vi "HFRR ADV v10.vi"() -> ()   [LabVIEW 2025] (continued)
                    n423 = Fract/Exp String To Number(string=w685) -> (number=w684:dbl)  [unwired: 3 in, 1 out]
                    n424 = local write "Average"(w684) -> ()
                  }
                }
              }
              frame True {
                w723 = 1000.0 ("y")
                w729 = 0.0 ("default (0 DBL)")
                n425 = Match Pattern(string=w735, regular expression=" \"width_px\":") -> (after substring=w733:string)  [unwired: 1 in, 3 out]
                n426 = Match Pattern(string=w733, regular expression="\"height_px\":") -> (before substring=w731:string, after substring=w730:string)  [unwired: 1 in, 2 out]
                n427 = Fract/Exp String To Number(string=w731, default (0 dbl)=w729) -> (number=w728:dbl)  [unwired: 2 in, 1 out]
                n428 = Fract/Exp String To Number(string=w730, default (0 dbl)=w729) -> (number=w727:dbl)  [unwired: 2 in, 1 out]
                n429 = Multiply(x=w728, y=w726) -> (x*y=w725:dbl)
                n430 = Multiply(x=w727, y=w726) -> (x*y=w724:dbl)
                n431 = Multiply(x=w725, y=w723) -> (x*y=w709:dbl)
                n432 = Multiply(x=w724, y=w723) -> (x*y=w707:dbl)
                n433 = Add(x=w709, y=w707) -> (x+y=w721:dbl)
                n434 = property on="Major Axis" class="DigNum (strict)"("Caption.Text"="Major Axis") -> ()  [unwired: 2 in, 2 out]
                n435 = property on="Minor Axis" class="DigNum (strict)"("Caption.Text"="Minor Axis") -> ()  [unwired: 2 in, 2 out]
                n436 = property on="Average" class="DigNum (strict)"("Caption.Text"="Average") -> ()  [unwired: 2 in, 2 out]
                n437 = Divide(x=w721, y=2.0) -> (x/y=w705:dbl)
                n438 = Bundle By Name(cluster=w722, "major"=w709, "minor"=w707, "average"=w705) -> (w719:cluster{"major":dbl, "minor":dbl, "average":dbl})
                n439 = Number To Fractional String(number=w707, precision (6)=i16 1) -> (F-format string=w714:string)  [unwired: 2 in]
                n440 = Number To Fractional String(number=w705, precision (6)=i16 1) -> (F-format string=w715:string)  [unwired: 2 in]
                n441 = Number To Fractional String(number=w709, precision (6)=i16 1) -> (F-format string=w713:string)  [unwired: 2 in]
                n442 = Fract/Exp String To Number(string=w714) -> (number=w706:dbl)  [unwired: 3 in, 1 out]
                n443 = Fract/Exp String To Number(string=w715) -> (number=w704:dbl)  [unwired: 3 in, 1 out]
                n444 = Fract/Exp String To Number(string=w713) -> (number=w708:dbl)  [unwired: 3 in, 1 out]
                n445 = local write "Major Axis"(w708) -> ()
                n446 = local write "Average"(w704) -> ()
                n447 = local write "Minor Axis"(w706) -> ()
              }
            }
            n448 = case shown="\"Measrument\", Default" w622 {
              tunnel: w625 -> [w649 _]
              tunnel: w624 -> [w648 _]
              tunnel: [w645 w673] -> w623
              tunnel: w621 -> [w647 w673]
              tunnel: w620 -> [w646 _]
              frame "Measrument", Default {
                n449 = stacked-sequence {
                  tunnel: w649 -> [w666 _]
                  tunnel: w648 -> [w664 _]
                  tunnel: w647 -> [w662 _]
                  tunnel: w646 -> [w661 _]
                  tunnel: [w656 _] -> w645
                  frame #0 {
                    n450 = call "IMAGE ANALYSIS.vi"("Enum"=POST_ANALYSIS_ENUM."SAVE IMAGE", "error in"=w662, "IMAGE FILE PATH"=w661) -> ("error out"=w660:errorcluster)  [unwired: 7 in, 1 out]
                    n451 = call "Stall Data Flow.vim"("value in"=w660, "milliseconds to wait"=u32 1000) -> ("value out"=w651:errorcluster)  [unwired: 1 out]
                    n452 = local read "Test File List :"() -> (w668:string)
                    n453 = call "IMAGE ANALYSIS.vi"("Enum"=POST_ANALYSIS_ENUM."MINIMIZE UI", "error in"=w651) -> ("error out"=w658:errorcluster)  [unwired: 8 in, 1 out]
                    n454 = Bundle By Name(cluster=T21 {"File Name"="", "Test Method"="", "Operator"="", "Fuel Description"="", "Date and time"=""} ("Main Ref"), "File Name"=w668) -> (w669:T21)
                    n455 = call "Stall Data Flow.vim"("value in"=w658, "milliseconds to wait"=u32 1500) -> ("value out"=w653:errorcluster)  [unwired: 1 out]
                    n456 = call "duf file read.vi"("error in (no error)"=w653, "Main Ref"=w669) -> ("error out"=w667:errorcluster, "Main Ref 2"=w665:T21)  [unwired: 8 in]
                    n457 = call "DETECTION REPORT for manual.vi"("error in (no error)"=w667, "return value 3"=w664, "Image File Path"=w666, "Main Ref"=w665) -> ("error out"=w663:errorcluster)  [unwired: 7 in]
                    n458 = call <vilib>:"Clear Errors.vi"("error in (no error)"=w663) -> ("error out"=w654:errorcluster)  [unwired: 5 in, 1 out]
                    n459 = call "IMAGE ANALYSIS.vi"("Enum"=POST_ANALYSIS_ENUM."MINIMIZE UI", "error in"=w654) -> ("error out"=w656:errorcluster)  [unwired: 8 in, 1 out]
                  }
                  frame #1 {
                    n460 = local write "Main Tab"(T2."HOME" ("Main Tab")) -> ()
                    n461 = local write "Main Dashboard Buttons"(T1."Home" ("Main Dashboard Buttons")) -> ()
                  }
                }
              }
              frame "Calibrate" {
              }
            }
          }
          frame #2 {
            n462 = Not(x=w738) -> (.not. x?=w737:bool)
            n463 = local write "Confirm Measrurement"(w737) -> ()
            n464 = local read "Calibration Tab"() -> (w736:enum32{"Measrument", "Calibrate"})
            n465 = case shown="\"Measrument\", Default" w736 {
              frame "Measrument", Default {
                n466 = local write "Main Tab"(T2."HOME" ("Main Tab")) -> ()
              }
              frame "Calibrate" {
              }
            }
          }
        }
      }
    }
    n467 = local read "Humidity"() -> (w487:bool)
    n468 = local read "Save Change"() -> (w492:bool)
    n469 = local read "Calibrate"() -> (w493:bool)
    n470 = local read "Auto Start Test"() -> (w488:bool)
    n471 = case shown="True" w493 {
      selector: w493 -> [_ w600]
      frame False {
      }
      frame True {
        n472 = Not(x=w600) -> (.not. x?=w599:bool)
        n473 = local write "Calibrate"(w599) -> ()
        n474 = local write "Calibration Tab"(enum32{"Measrument", "Calibrate"}."Calibrate" ("Calibration Tab")) -> ()
      }
    }
    n475 = case shown="True" w492 {
      selector: w492 -> [_ w544]
      frame False {
      }
      frame True {
        n476 = stacked-sequence {
          tunnel: w544 -> [_ _ _ _ w598]
          frame #0 {
            n477 = call "IMAGE ANALYSIS.vi"("Enum"=POST_ANALYSIS_ENUM."HIDE UI") -> ()  [unwired: 9 in, 2 out]
          }
          frame #1 {
            n478 = local read "100x gain"() -> (w546:dbl)
            n479 = local read "10x Gain"() -> (w547:dbl)
            n480 = local read "5x Gain"() -> (w548:dbl)
            n481 = Number To Fractional String(number=w547, width (-)=i16 4, precision (6)=i16 7) -> (F-format string=w569:string)  [unwired: 1 in]
            n482 = Number To Fractional String(number=0.0, width (-)=i16 4, precision (6)=i16 7) -> (F-format string=w564:string)  [unwired: 1 in]
            n483 = Number To Fractional String(number=w546, width (-)=i16 4, precision (6)=i16 7) -> (F-format string=w552:string)  [unwired: 1 in]
            n484 = Number To Fractional String(number=w548, width (-)=i16 10 ("precision (6)"), precision (6)=i16 7) -> (F-format string=w578:string)  [unwired: 1 in]
            n485 = Concatenate Strings("[CH1]" ("string"), w578, " - 5x Gain" ("string"), "\r") -> (w568:string)
            n486 = Concatenate Strings("[CH2]" ("string"), w569, " - 10x Gain" ("string"), "\r") -> (w567:string)
            n487 = Concatenate Strings("[CH3]" ("string"), w564, " - 20x Gain" ("string"), "\r") -> (w558:string)
            n488 = Concatenate Strings("[CH4]" ("string"), w552, " - 100x Gain" ("string"), "\r") -> (w551:string)
            n489 = String To Path(string="C:\\LAB-IQ\\Image Calibrate v01.dcf") -> (path=w581:path)
            n490 = Concatenate Strings(w568, w567, w558, w551) -> (w566:string)
            n491 = call <vilib>:"Write Characters To File.vi"("append to file? (new file:F)"=FALSE, "character string"=w566, "file path (dialog if empty)"=w581) -> ()  [unwired: 2 in, 1 out]
          }
          frame #2 {
            n492 = String To Path(string="C:\\LAB-IQ\\Image Calibrate v01.dcf") -> (path=w584:path)
            n493 = Open/Create/Replace File ("Open File")(file path (use dialog)=w584) -> (refnum out=w585:refnum<file>)  [unwired: 5 in, 2 out]
            n494 = for {
              N: 4 -> [_]
              tunnel: w585 -> [w591]
              i -> [w587]
              n495 = Read from Text File ("Read File")(file (use dialog)=w591) -> (text=w592:string)  [unwired: 3 in, 3 out]
              n496 = String Subset(string=w592, offset (0)=6, length (rest)=10 ("length (rest)")) -> (substring=w588:string)
              n497 = Fract/Exp String To Number(string=w588) -> (number=w586:dbl)  [unwired: 3 in, 1 out]
              n498 = case shown="3" w587 {
                tunnel: w586 -> [w593 w594 _ w595 _]
                frame 0 {
                  n499 = local write "5x Gain"(w593) -> ()
                }
                frame 1 {
                  n500 = local write "10x Gain"(w594) -> ()
                }
                frame 2 {
                }
                frame 3 {
                  n501 = local write "100x gain"(w595) -> ()
                }
                frame 4, Default {
                }
              }
            }
          }
          frame #3 {
            n502 = call "IMAGE ANALYSIS.vi"("Enum"=POST_ANALYSIS_ENUM."SHOW UI") -> ()  [unwired: 9 in, 2 out]
          }
          frame #4 {
            n503 = Not(x=w598) -> (.not. x?=w597:bool)
            n504 = local write "Save Change"(w597) -> ()
          }
        }
      }
    }
    n505 = case shown="False" w488 {
      tunnel: w487 -> [w514 _]
      frame False {
        n506 = case shown="True" w514 {
          frame False {
          }
          frame True {
            n507 = local read "Set Humidity:"() -> (w518:dbl)
            n508 = local read "Set Humidity:"() -> (w521:dbl)
            n509 = local read "Humidity ( %RH )"() -> (w522:dbl)
            n510 = Subtract(x=w518, y=1.0) -> (x-y=w516:dbl)
            n511 = Add(x=w521, y=1.0) -> (x+y=w517:dbl)
            n512 = In Range and Coerce(upper limit=w517, x=w522, lower limit=w516) -> (In Range?=w515:bool)  [unwired: 1 out]
            n513 = case shown="True" w515 {
              frame False {
              }
              frame True {
                n514 = case shown="True" "Manual Humididty Reached" {
                  selector: "Manual Humididty Reached" -> [_ w525]
                  frame False {
                  }
                  frame True {
                    n515 = Not(x=w525) -> (.not. x?=w524:bool)
                    n516 = local write "Manual Humididty Reached"(w524) -> ()
                    n517 = local read "EVENT LOG"() -> (w527:string)
                    n518 = call "Event Log.vi"("Content"="Target Humidity reached", "EVENT LOG"=w527) -> ("EVENT LOG"=w526:string)  [unwired: 8 in, 1 out]
                    n519 = local write "EVENT LOG"(w526) -> ()
                  }
                }
              }
            }
          }
        }
      }
      frame True {
        n520 = local write "Manual Humididty Reached"(TRUE ("Manual Humididty Reached")) -> ()
      }
    }
    n521 = local read "Cap Live Image"() -> (w508:bool)
    n522 = local read "SCAR MEASURMENT"() -> (w511:enum32{"Auto Scar", "Manual Scar"})
    n523 = Wait (ms)(milliseconds to wait=u32 250) -> ()  [unwired: 1 out]
    n524 = Equal?(x=w511, y=enum32{"Auto Scar", "Manual Scar"}."Manual Scar" ("SCAR MEASURMENT")) -> (x = y?=w509:bool)
    n525 = And(x=w509, y=w508) -> (x .and. y?=w507:bool)
    n526 = case shown="True" w507 {
      selector: w507 -> [_ w817]
      frame False {
      }
      frame True {
        n527 = stacked-sequence {
          tunnel: [_ _ _ w832 _] -> _
          tunnel: w817 -> [_ _ _ _ w838]
          frame #0 {
            w818 = 0.0
            n528 = local write "Major Axis"(w818) -> ()
            n529 = local write "Minor Axis"(w818) -> ()
            n530 = local write "Average"(w818) -> ()
          }
          frame #1 {
            n531 = call "CAMERA LIVE FEED FGV.vi"("Enum - Menu"=CAMERA_LIVE_FEED_ENUM."CAMERA MINIMIZE") -> ()  [unwired: 9 in, 2 out]
          }
          frame #2 {
            n532 = local read "FILE 3"() -> (w826:string)
            n533 = call <vilib>:"Trim Whitespace.vi"("string"="C:\\LAB-IQ\\images\\") -> ("trimmed string"=w828:string)  [unwired: 1 in]
            n534 = String To Path(string=w828) -> (path=w827:path)
            n535 = Concatenate Strings(w826, ".png" ("string")) -> (w825:string)
            n536 = Build Path(base path=w827, name or relative path=w825) -> (appended path=w823:path)
            n537 = Path To String(path=w823) -> (string=w822:string)
            n538 = call "CAMERA LIVE FEED FGV.vi"("Enum - Menu"=CAMERA_LIVE_FEED_ENUM."CAMERA SAVE", "Image Path"=w822) -> ("error out"=w820:errorcluster)  [unwired: 8 in, 1 out]
            n539 = case shown="No Error" w820 {
              frame No Error {
                n540 = One Button Dialog(message="Image saved successfully") -> ()  [unwired: 1 in, 1 out]
              }
              frame Error {
              }
            }
          }
          frame #3 {
            n541 = call "LIST FILE NAMES.vi"() -> ("error out"=w834:errorcluster, "filenames"=w831:string[])  [unwired: 10 in]
            n542 = call "IMAGE ANALYSIS.vi"("Enum"=POST_ANALYSIS_ENUM."SHOW UI", "error in"=w834) -> ("error out"=w832:errorcluster)  [unwired: 8 in, 1 out]
            n543 = property on="Test File List :" class="CmbBox"("Strings[]"=w831) -> ()  [unwired: 2 in, 2 out]
          }
          frame #4 {
            (unwired) T22."Report" ("Main Dashboard Buttons")
            n544 = Not(x=w838) -> (.not. x?=w837:bool)
            n545 = local write "Zoom Factore"(0.0 ("Zoom Factore")) -> ()
            n546 = local write "Cap Live Image"(w837) -> ()
            n547 = local write "Main Tab"(T2."Adv Scar Report" ("Main Tab")) -> ()
            n548 = property on="Cap Live Image" class="Bool (strict)"("BoolText.Text"="Capture Image" ("Boolean Text.Text")) -> ()  [unwired: 2 in, 2 out]
            n549 = local write "Main Dashboard Buttons"(T1."Report" ("Main Dashboard Buttons")) -> ()
          }
        }
      }
    }
    n550 = local read "change Gain"() -> (w491:bool)
    n551 = local read "Back Square"() -> (w490:bool)
    n552 = case shown="True" w491 {
      selector: w491 -> [_ w535]
      frame False {
      }
      frame True {
        n553 = stacked-sequence {
          tunnel: w535 -> [_ w543]
          frame #0 {
            n554 = local read "Actual (µm)"() -> (w539:dbl)
            n555 = local read "Pixel Value"() -> (w538:dbl)
            n556 = local read "Magnification :"() -> (w537:string)
            n557 = Divide(x=w539, y=w538) -> (x/y=w536:dbl)
            n558 = case shown="\"10x\"" w537 {
              tunnel: w536 -> [w540 w541]
              frame "10x" {
                n559 = local write "10x Gain"(w540) -> ()
              }
              frame "5x", Default {
                n560 = local write "5x Gain"(w541) -> ()
              }
            }
          }
          frame #1 {
            n561 = Not(x=w543) -> (.not. x?=w542:bool)
            n562 = local write "change Gain"(w542) -> ()
          }
        }
      }
    }
    n563 = case shown="True" w490 {
      selector: w490 -> [_ w533]
      frame False {
      }
      frame True {
        n564 = Not(x=w533) -> (.not. x?=w532:bool)
        n565 = local write "Back Square"(w532) -> ()
        n566 = local write "Calibration Tab"(enum32{"Measrument", "Calibrate"}."Measrument" ("Calibration Tab")) -> ()
      }
    }
    n567 = local read "Rectangle Tool"() -> (w502:bool)
    n568 = local read "Clear ROI Tool"() -> (w501:bool)
    n569 = local read "Open Image"() -> (w506:bool)
    n570 = local read "line tool"() -> (w503:bool)
    n571 = local read "OUT"() -> (w504:bool)
    n572 = local read "In"() -> (w505:bool)
    n573 = case shown="True" w506 {
      selector: w506 -> [_ w805]
      tunnel: [w801 w807] -> _
      tunnel: w496 -> [w801 w806]
      frame False {
      }
      frame True {
        n574 = Not(x=w805) -> (.not. x?=w804:bool)
        n575 = local write "Open Image"(w804) -> ()
        n576 = call "IMAGE ANALYSIS.vi"("Enum"=POST_ANALYSIS_ENUM."HIDE UI", "error in"=w806) -> ("error out"=w814:errorcluster)  [unwired: 8 in, 1 out]
        n577 = call "File Dialog"("start path"=path "C:/LAB-IQ/images", "error in"=w814) -> ("selected path"=w803:path, "error out"=w812:errorcluster)  [unwired: 10 in, 2 out]
        "Image path  2" <- w803
        n578 = call <vilib>:"Clear Errors.vi"("error in (no error)"=w812) -> ("error out"=w811:errorcluster)  [unwired: 5 in, 1 out]
        n579 = call "IMAGE ANALYSIS.vi"("Enum"=POST_ANALYSIS_ENUM."OPEN FILE", "error in"=w811, "File Path"=w803) -> ("error out"=w810:errorcluster)  [unwired: 7 in, 1 out]
        n580 = call <vilib>:"Clear Errors.vi"("error in (no error)"=w810) -> ("error out"=w809:errorcluster)  [unwired: 5 in, 1 out]
        n581 = call "IMAGE ANALYSIS.vi"("Enum"=POST_ANALYSIS_ENUM."SHOW UI", "error in"=w809) -> ("error out"=w807:errorcluster)  [unwired: 8 in, 1 out]
        n582 = local write "Zoom Factore"(100.0 ("Zoom Factore")) -> ()
      }
    }
    n583 = case shown="True" w504 {
      selector: w504 -> [_ w786]
      tunnel: w496 -> [w783 w791]
      tunnel: [w783 w785] -> _
      frame False {
      }
      frame True {
        n584 = Not(x=w786) -> (.not. x?=w784:bool)
        n585 = local read "Zoom Factore"() -> (w789:dbl)
        n586 = local write "OUT"(w784) -> ()
        n587 = call "IMAGE ANALYSIS.vi"("Enum"=POST_ANALYSIS_ENUM."ZOOM OUT", "error in"=w791) -> ("error out"=w785:errorcluster)  [unwired: 8 in, 1 out]
        n588 = Divide(x=w789, y=1.2) -> (x/y=w787:dbl)
        n589 = local write "Zoom Factore"(w787) -> ()
      }
    }
    n590 = case shown="True" w505 {
      selector: w505 -> [_ w795]
      tunnel: w496 -> [w792 w800]
      tunnel: [w792 w793] -> _
      frame False {
      }
      frame True {
        n591 = Not(x=w795) -> (.not. x?=w794:bool)
        n592 = local read "Zoom Factore"() -> (w798:dbl)
        n593 = local write "In"(w794) -> ()
        n594 = call "IMAGE ANALYSIS.vi"("Enum"=POST_ANALYSIS_ENUM."ZOOM IN", "error in"=w800) -> ("error out"=w793:errorcluster)  [unwired: 8 in, 1 out]
        n595 = Multiply(x=w798, y=1.2) -> (x*y=w796:dbl)
        n596 = local write "Zoom Factore"(w796) -> ()
      }
    }
    n597 = case shown="True" w501 {
      selector: w501 -> [_ w767]
      tunnel: w496 -> [w765 w769]
      tunnel: [w765 w768] -> _
      frame False {
      }
      frame True {
        n598 = Not(x=w767) -> (.not. x?=w766:bool)
        n599 = local write "Clear ROI Tool"(w766) -> ()
        n600 = call "IMAGE ANALYSIS.vi"("Enum"=POST_ANALYSIS_ENUM."CLEAR ROI", "error in"=w769) -> ("error out"=w768:errorcluster)  [unwired: 8 in, 1 out]
      }
    }
    n601 = case shown="True" w503 {
      selector: w503 -> [_ w779]
      tunnel: w496 -> [w777 w782]
      tunnel: [w777 w780] -> _
      frame False {
      }
      frame True {
        n602 = Not(x=w779) -> (.not. x?=w778:bool)
        n603 = local write "line tool"(w778) -> ()
        n604 = call "IMAGE ANALYSIS.vi"("Enum"=POST_ANALYSIS_ENUM."DRAW LINE", "error in"=w782) -> ("error out"=w780:errorcluster)  [unwired: 8 in, 1 out]
      }
    }
    n605 = case shown="True" w502 {
      selector: w502 -> [_ w773]
      tunnel: w496 -> [w771 w775]
      tunnel: [w771 w774] -> _
      frame False {
      }
      frame True {
        n606 = Not(x=w773) -> (.not. x?=w772:bool)
        n607 = local write "Rectangle Tool"(w772) -> ()
        n608 = call "IMAGE ANALYSIS.vi"("Enum"=POST_ANALYSIS_ENUM."DRAW REC", "error in"=w775) -> ("error out"=w774:errorcluster)  [unwired: 8 in, 1 out]
      }
    }
    n609 = local read "SCAR MEASURMENT"() -> (w489:enum32{"Auto Scar", "Manual Scar"})
    n610 = local read "Fit to Screen Tool"() -> (w498:bool)
    n611 = local read "Resize Tool"() -> (w497:bool)
    n612 = case shown="\"Manual Scar\", Default" w489 {
      frame "Auto Scar" {
        n613 = property on="Cap Live Image" class="Bool (strict)"("BoolText.Text"="Report" ("Boolean Text.Text")) -> ()  [unwired: 2 in, 2 out]
      }
      frame "Manual Scar", Default {
        n614 = property on="Cap Live Image" class="Bool (strict)"("BoolText.Text"="Save Image" ("Boolean Text.Text")) -> ()  [unwired: 2 in, 2 out]
      }
    }
    n615 = local read "ROI Color Tool"() -> (w499:bool)
    n616 = local read "Pan Tool"() -> (w500:bool)
    n617 = case shown="True" w500 {
      selector: w500 -> [_ w761]
      tunnel: w496 -> [w759 w763]
      tunnel: [w759 w762] -> _
      frame False {
      }
      frame True {
        n618 = Not(x=w761) -> (.not. x?=w760:bool)
        n619 = call "IMAGE ANALYSIS.vi"("Enum"=POST_ANALYSIS_ENUM."PAN", "error in"=w763) -> ("error out"=w762:errorcluster)  [unwired: 8 in, 1 out]
        n620 = local write "Pan Tool"(w760) -> ()
      }
    }
    n621 = case shown="True" w497 {
      selector: w497 -> [_ w745]
      tunnel: w496 -> [w740 w742]
      tunnel: [w740 w741] -> _
      frame False {
      }
      frame True {
        n622 = Not(x=w745) -> (.not. x?=w744:bool)
        n623 = local write "Resize Tool"(w744) -> ()
        n624 = call "IMAGE ANALYSIS.vi"("Enum"=POST_ANALYSIS_ENUM."RESIZE MODE", "error in"=w742) -> ("error out"=w741:errorcluster)  [unwired: 8 in, 1 out]
      }
    }
    n625 = case shown="True" w498 {
      selector: w498 -> [_ w750]
      tunnel: [w746 w751] -> _
      tunnel: w496 -> [w746 w749]
      frame False {
      }
      frame True {
        n626 = Not(x=w750) -> (.not. x?=w748:bool)
        n627 = local write "Zoom Factore"(100.0 ("Zoom Factore")) -> ()
        n628 = local write "Fit to Screen Tool"(w748) -> ()
        n629 = call "IMAGE ANALYSIS.vi"("Enum"=POST_ANALYSIS_ENUM."FIT", "error in"=w749) -> ("error out"=w751:errorcluster)  [unwired: 8 in, 1 out]
      }
    }
    n630 = case shown="True" w499 {
      selector: w499 -> [_ w756]
      tunnel: [w753 w757] -> _
      tunnel: w496 -> [w753 w754]
      frame False {
      }
      frame True {
        n631 = Not(x=w756) -> (.not. x?=w755:bool)
        n632 = local write "ROI Color Tool"(w755) -> ()
        n633 = call "IMAGE ANALYSIS.vi"("Enum"=POST_ANALYSIS_ENUM."SET ROI COLOR", "error in"=w754) -> ("error out"=w757:errorcluster)  [unwired: 8 in, 1 out]
      }
    }
    n634 = local read "Quit"() -> (w513:bool)
  }
  n635 = local write "USERNAME"(w28) -> ()
  n636 = local write "Main Tab"(T2."HOME" ("Main Tab")) -> ()
  n637 = local write "USER ID"(w28) -> ()
  n638 = property on="Auto Scar Check  2" class="Clust (strict)"("Visible"=w9) -> (error out=w13:errorcluster)  [unwired: 2 in, 1 out]
  n639 = property on="Quit" class="Bool (strict)"("Value"=FALSE ("Quit")) -> (error out=w30:errorcluster)  [unwired: 2 in, 1 out]
  n640 = while {
    stop <- w841 stop-if-true
    n641 = local read "Image Path"() -> (w844:path)
    n642 = local read "Print 3"() -> (w847:bool)
    n643 = Equal?(x=w844, y=path "") -> (x = y?=w843:bool)
    n644 = Not(x=w843) -> (.not. x?=w842:bool)
    n645 = property on="Print 3" class="Bool (strict)"("Visible"=w842) -> ()  [unwired: 2 in, 2 out]
    n646 = case shown="True" w847 {
      frame False {
        n647 = local write "Rd"(TRUE ("Boolean 7")) -> ()
      }
      frame True {
        n648 = flat-sequence {
          tunnel: [w887] -> w855
          tunnel: [w874] -> w853
          tunnel: [w884] -> w849
          tunnel: w855 -> [w896]
          tunnel: [w896] -> w854
          tunnel: w853 -> [w895]
          tunnel: [w895] -> w852
          tunnel: [w893] -> w851
          tunnel: [w892] -> w850
          tunnel: w849 -> [w892]
          tunnel: w854 -> [w898]
          tunnel: w852 -> [w899]
          tunnel: w851 -> [_]
          tunnel: w850 -> [w897]
          frame #0 {
            n649 = case shown="True" "Rd" {
              frame False {
              }
              frame True {
                n650 = while {
                  tunnel: "abcdefABCDEF" ("string 2") -> [w866]
                  shift-right: [w864] -> w858
                  shift-left: "" -> [w863]
                  i -> [w873]
                  stop <- w872 stop-if-true
                  n651 = Random Number (0-1)() -> (number: 0 to 1=w867:dbl)
                  n652 = Multiply(x=w867, y=62.0) -> (x*y=w869:dbl)
                  n653 = Decrement(x="Length 2") -> (x-1=w862:i16)
                  n654 = To Word Integer(number=w869) -> (16bit integer=w870:i16)
                  n655 = String Subset(string=w866, offset (0)=w870, length (rest)=1 ("length (rest)")) -> (substring=w865:string)
                  n656 = Greater Or Equal?(x=w873, y=w862) -> (x >= y?=w872:bool)
                  n657 = Concatenate Strings(w865, w863) -> (w864:string)
                }
                "String 10" <- w858
                n658 = local write "Rd"(FALSE ("Boolean 7")) -> ()
              }
            }
          }
          frame #1 {
            w885 = "_resized.jpg" ("command line")
            (unwired) ".jpg -resize 320x240 " ("string")
            (unwired) "Choose an Image File" ("prompt")
            # "-resize 1798x425"
            n659 = local read "Image Path"() -> (w879:path)
            n660 = Strip Path(path=w879) -> (stripped path=w874:path, name=w875:string)
            n661 = Match Pattern(string=w875, regular expression=".jpg") -> (before substring=→"before substring 2":string, after substring=→"after substring":string)  [unwired: 1 in, 2 out]
            n662 = Match Pattern(string=w875, regular expression="\\") -> (before substring=w881:string)  [unwired: 1 in, 3 out]
            n663 = Match Pattern(string=w881, regular expression=".jpg") -> (before substring=w880:string)  [unwired: 1 in, 3 out]
            n664 = Concatenate Strings("cmd /c convert " ("string"), w880, ".jpg -resize 320x240  " ("command line"), w880, w885) -> (w888:string)
            n665 = call <vilib>:"System Exec.vi"("run minimized? (F)"=TRUE, "wait until completion? (T)"=TRUE, "working directory"=w874, "command line"=w888) -> ("error out"=w887:errorcluster)  [unwired: 4 in, 3 out]
            "error out 2" <- w887
            n666 = Concatenate Strings(w880, w885) -> (w884:string)
          }
          frame #2 {
            n667 = Wait (ms)(milliseconds to wait=u32 2000 ("millisecond timer value")) -> (millisecond timer value=w893:u32)
          }
          frame #3 {
            n668 = case shown="No Error" w898 {
              tunnel: w899 -> [w902 _]
              tunnel: w897 -> [w900 _]
              frame No Error {
                (unwired) ".jpg" ("string")
                n669 = Path To String(path=w902) -> (string=w906:string)
                n670 = Concatenate Strings(w906, "\\" ("string"), w900) -> (w905:string)
                n671 = String To Path(string=w905) -> (path=w904:path)
                n672 = call <vilib>:"Read JPEG File.vi"("path to JPEG file"=w904) -> ("image data"=w908:T14)  [unwired: 8 in, 2 out]
                "image data" <- w908
                n673 = local write "Print 3"(FALSE ("Print 2")) -> ()
                n674 = call <vilib>:"Draw Flattened Pixmap.vi"("image data"=w908) -> ("new picture"=→"new picture":picture)  [unwired: 8 in]
              }
              frame Error {
              }
            }
          }
        }
      }
    }
    n675 = Wait (ms)(milliseconds to wait=u32 20 ("millisecond timer value")) -> ()  [unwired: 1 out]
    n676 = local read "Quit"() -> (w841:bool)
  }
  n677 = property on="Service Password Log" class="Str"("Visible"=w9) -> ()  [unwired: 2 in, 2 out]
  n678 = property on="Password 3" class="Clust (strict)"("Visible"=w9) -> ()  [unwired: 2 in, 2 out]
  n679 = while {
    tunnel: w30 -> [_]
    tunnel: w13 -> [_]
    stop <- w939 stop-if-true
    # "New Adv Logics"
    n680 = local read "Main Tab"() -> (w937:T2)
    n681 = local read "Sign In"() -> (w936:bool)
    n682 = local read "Main Tab"() -> (w918:T2)
    n683 = case shown="\"About\"" w918 {
      frame "HOME", Default {
        n684 = local read "LIVE FEED MIN TEMP"() -> (w1062:bool)
        n685 = local write "LIVE FEED MAX TEMP"(TRUE ("LIVE FEED MAX TEMP")) -> ()
        n686 = local read "CAMERA ROI MIN TEMP"() -> (w1060:bool)
        n687 = case shown="True" w1062 {
          selector: w1062 -> [_ w1069]
          frame False {
          }
          frame True {
            n688 = Not(x=w1069) -> (.not. x?=w1068:bool)
            n689 = local write "LIVE FEED MIN TEMP"(w1068) -> ()
            n690 = call "CAMERA LIVE FEED FGV.vi"("Enum - Menu"=CAMERA_LIVE_FEED_ENUM."CAMERA MINIMIZE") -> ()  [unwired: 9 in, 2 out]
          }
        }
        n691 = case shown="True" w1060 {
          selector: w1060 -> [_ w1066]
          frame False {
          }
          frame True {
            n692 = Not(x=w1066) -> (.not. x?=w1065:bool)
            n693 = local write "CAMERA ROI MIN TEMP"(w1065) -> ()
            n694 = call "IMAGE ANALYSIS.vi"("Enum"=POST_ANALYSIS_ENUM."MINIMIZE UI") -> ()  [unwired: 9 in, 2 out]
          }
        }
        n695 = local write "CAMERA ROI MAX TEMP"(TRUE ("CAMERA ROI MAX TEMP")) -> ()
      }
      frame "Test Setup" {
        n696 = local read "LIVE FEED MIN TEMP"() -> (w1072:bool)
        n697 = local read "CAMERA ROI MIN TEMP"() -> (w1070:bool)
        n698 = local write "LIVE FEED MAX TEMP"(TRUE ("LIVE FEED MAX TEMP")) -> ()
        n699 = case shown="True" w1072 {
          selector: w1072 -> [_ w1079]
          frame False {
          }
          frame True {
            n700 = Not(x=w1079) -> (.not. x?=w1078:bool)
            n701 = local write "LIVE FEED MIN TEMP"(w1078) -> ()
            n702 = call "CAMERA LIVE FEED FGV.vi"("Enum - Menu"=CAMERA_LIVE_FEED_ENUM."CAMERA MINIMIZE") -> ()  [unwired: 9 in, 2 out]
          }
        }
        n703 = case shown="True" w1070 {
          selector: w1070 -> [_ w1076]
          frame False {
          }
          frame True {
            n704 = Not(x=w1076) -> (.not. x?=w1075:bool)
            n705 = local write "CAMERA ROI MIN TEMP"(w1075) -> ()
            n706 = call "IMAGE ANALYSIS.vi"("Enum"=POST_ANALYSIS_ENUM."MINIMIZE UI") -> ()  [unwired: 9 in, 2 out]
          }
        }
        n707 = local write "CAMERA ROI MAX TEMP"(TRUE ("CAMERA ROI MAX TEMP")) -> ()
      }
      frame "Acquire" {
        n708 = local read "LIVE FEED MIN TEMP"() -> (w1082:bool)
        n709 = local write "LIVE FEED MAX TEMP"(TRUE ("LIVE FEED MAX TEMP")) -> ()
        n710 = local read "CAMERA ROI MIN TEMP"() -> (w1080:bool)
        n711 = case shown="True" w1082 {
          selector: w1082 -> [_ w1089]
          frame False {
          }
          frame True {
            n712 = Not(x=w1089) -> (.not. x?=w1088:bool)
            n713 = local write "LIVE FEED MIN TEMP"(w1088) -> ()
            n714 = call "CAMERA LIVE FEED FGV.vi"("Enum - Menu"=CAMERA_LIVE_FEED_ENUM."CAMERA MINIMIZE") -> ()  [unwired: 9 in, 2 out]
          }
        }
        n715 = case shown="True" w1080 {
          selector: w1080 -> [_ w1086]
          frame False {
          }
          frame True {
            n716 = Not(x=w1086) -> (.not. x?=w1085:bool)
            n717 = local write "CAMERA ROI MIN TEMP"(w1085) -> ()
            n718 = call "IMAGE ANALYSIS.vi"("Enum"=POST_ANALYSIS_ENUM."MINIMIZE UI") -> ()  [unwired: 9 in, 2 out]
          }
        }
        n719 = local write "CAMERA ROI MAX TEMP"(TRUE ("CAMERA ROI MAX TEMP")) -> ()
      }
      frame "Adv Scar" {
        n720 = local read "CAMERA ROI MIN TEMP"() -> (w1090:bool)
        n721 = case shown="True" "LIVE FEED MAX TEMP" {
          selector: "LIVE FEED MAX TEMP" -> [_ w1102]
          frame False {
          }
          frame True {
            n722 = Not(x=w1102) -> (.not. x?=w1101:bool)
            n723 = local write "LIVE FEED MAX TEMP"(w1101) -> ()
            n724 = call "CAMERA LIVE FEED FGV.vi"("Enum - Menu"=CAMERA_LIVE_FEED_ENUM."CAMERA RESTORE") -> ("error out"=w1097:errorcluster)  [unwired: 9 in, 1 out]
            n725 = call "LIST FILE NAMES.vi"("error in (no error)"=w1097) -> ("error out"=w1098:errorcluster, "filenames"=w1099:string[])  [unwired: 9 in]
            n726 = property on="FILE 3" class="CmbBox"(error in=w1098, "Strings[]"=w1099) -> ()  [unwired: 1 in, 2 out]
          }
        }
        n727 = case shown="True" w1090 {
          selector: w1090 -> [_ w1096]
          frame False {
          }
          frame True {
            n728 = Not(x=w1096) -> (.not. x?=w1095:bool)
            n729 = local write "CAMERA ROI MIN TEMP"(w1095) -> ()
            n730 = call "IMAGE ANALYSIS.vi"("Enum"=POST_ANALYSIS_ENUM."MINIMIZE UI") -> ()  [unwired: 9 in, 2 out]
          }
        }
        n731 = local write "CAMERA ROI MAX TEMP"(TRUE ("CAMERA ROI MAX TEMP")) -> ()
        "LIVE FEED MIN TEMP" <- TRUE ("LIVE FEED MIN TEMP")
      }
      frame "Adv Scar Report" {
        n732 = local read "CAMERA ROI MAX TEMP"() -> (w1103:bool)
        n733 = local read "LIVE FEED MIN TEMP"() -> (w1105:bool)
        n734 = local write "LIVE FEED MAX TEMP"(TRUE ("LIVE FEED MAX TEMP")) -> ()
        n735 = case shown="True" w1105 {
          selector: w1105 -> [_ w1114]
          frame False {
          }
          frame True {
            n736 = Not(x=w1114) -> (.not. x?=w1113:bool)
            n737 = local write "LIVE FEED MIN TEMP"(w1113) -> ()
            n738 = call "CAMERA LIVE FEED FGV.vi"("Enum - Menu"=CAMERA_LIVE_FEED_ENUM."CAMERA MINIMIZE") -> ()  [unwired: 9 in, 2 out]
          }
        }
        n739 = case shown="True" w1103 {
          selector: w1103 -> [_ w1111]
          frame False {
          }
          frame True {
            n740 = Not(x=w1111) -> (.not. x?=w1109:bool)
            n741 = local write "CAMERA ROI MAX TEMP"(w1109) -> ()
            n742 = call "IMAGE ANALYSIS.vi"("Enum"=POST_ANALYSIS_ENUM."SHOW UI") -> ("error out"=w1108:errorcluster)  [unwired: 9 in, 1 out]
            n743 = call "LIST FILE NAMES.vi"("error in (no error)"=w1108) -> ("filenames"=w1107:string[])  [unwired: 9 in, 1 out]
            n744 = property on="Test File List :" class="CmbBox"("Strings[]"=w1107) -> ()  [unwired: 2 in, 2 out]
          }
        }
        n745 = local write "CAMERA ROI MIN TEMP"(TRUE ("CAMERA ROI MIN TEMP")) -> ()
      }
      frame "Compare Files" {
        n746 = local read "LIVE FEED MIN TEMP"() -> (w1117:bool)
        n747 = local write "LIVE FEED MAX TEMP"(TRUE ("LIVE FEED MAX TEMP")) -> ()
        n748 = local read "CAMERA ROI MIN TEMP"() -> (w1115:bool)
        n749 = case shown="True" w1117 {
          selector: w1117 -> [_ w1124]
          frame False {
          }
          frame True {
            n750 = Not(x=w1124) -> (.not. x?=w1123:bool)
            n751 = local write "LIVE FEED MIN TEMP"(w1123) -> ()
            n752 = call "CAMERA LIVE FEED FGV.vi"("Enum - Menu"=CAMERA_LIVE_FEED_ENUM."CAMERA MINIMIZE") -> ()  [unwired: 9 in, 2 out]
          }
        }
        n753 = case shown="True" w1115 {
          selector: w1115 -> [_ w1121]
          frame False {
          }
          frame True {
            n754 = Not(x=w1121) -> (.not. x?=w1120:bool)
            n755 = local write "CAMERA ROI MIN TEMP"(w1120) -> ()
            n756 = call "IMAGE ANALYSIS.vi"("Enum"=POST_ANALYSIS_ENUM."MINIMIZE UI") -> ()  [unwired: 9 in, 2 out]
          }
        }
        n757 = local write "CAMERA ROI MAX TEMP"(TRUE ("CAMERA ROI MAX TEMP")) -> ()
      }
      frame "About" {
        n758 = local read "LIVE FEED MIN TEMP"() -> (w1127:bool)
        n759 = local write "LIVE FEED MAX TEMP"(TRUE ("LIVE FEED MAX TEMP")) -> ()
        n760 = local read "CAMERA ROI MIN TEMP"() -> (w1126:bool)
        n761 = case shown="True" w1127 {
          selector: w1127 -> [_ w1134]
          frame False {
          }
          frame True {
            n762 = Not(x=w1134) -> (.not. x?=w1133:bool)
            n763 = local write "LIVE FEED MIN TEMP"(w1133) -> ()
            n764 = call "CAMERA LIVE FEED FGV.vi"("Enum - Menu"=CAMERA_LIVE_FEED_ENUM."CAMERA MINIMIZE") -> ()  [unwired: 9 in, 2 out]
          }
        }
        n765 = case shown="True" w1126 {
          selector: w1126 -> [_ w1131]
          frame False {
          }
          frame True {
            n766 = Not(x=w1131) -> (.not. x?=w1130:bool)
            n767 = local write "CAMERA ROI MIN TEMP"(w1130) -> ()
            n768 = call "IMAGE ANALYSIS.vi"("Enum"=POST_ANALYSIS_ENUM."MINIMIZE UI") -> ()  [unwired: 9 in, 2 out]
          }
        }
        n769 = local write "CAMERA ROI MAX TEMP"(TRUE ("CAMERA ROI MIN TEMP")) -> ()
      }
      frame "Advance" {
        n770 = local read "LIVE FEED MIN TEMP"() -> (w1137:bool)
        n771 = local write "LIVE FEED MAX TEMP"(TRUE ("LIVE FEED MAX TEMP")) -> ()
        n772 = local read "CAMERA ROI MIN TEMP"() -> (w1135:bool)
        n773 = case shown="True" w1137 {
          selector: w1137 -> [_ w1144]
          frame False {
          }
          frame True {
            n774 = Not(x=w1144) -> (.not. x?=w1143:bool)
            n775 = local write "LIVE FEED MIN TEMP"(w1143) -> ()
            n776 = call "CAMERA LIVE FEED FGV.vi"("Enum - Menu"=CAMERA_LIVE_FEED_ENUM."CAMERA MINIMIZE") -> ()  [unwired: 9 in, 2 out]
          }
        }
        n777 = local write "CAMERA ROI MAX TEMP"(TRUE ("CAMERA ROI MAX TEMP")) -> ()
        n778 = case shown="True" w1135 {
          selector: w1135 -> [_ w1141]
          frame False {
          }
          frame True {
            n779 = Not(x=w1141) -> (.not. x?=w1140:bool)
            n780 = local write "CAMERA ROI MIN TEMP"(w1140) -> ()
            n781 = call "IMAGE ANALYSIS.vi"("Enum"=POST_ANALYSIS_ENUM."MINIMIZE UI") -> ()  [unwired: 9 in, 2 out]
          }
        }
      }
      frame "Mooha" {
        n782 = local read "LIVE FEED MIN TEMP"() -> (w1147:bool)
        n783 = local write "LIVE FEED MAX TEMP"(TRUE ("LIVE FEED MAX TEMP")) -> ()
        n784 = local read "CAMERA ROI MIN TEMP"() -> (w1145:bool)
        n785 = case shown="True" w1147 {
          selector: w1147 -> [_ w1154]
          frame False {
          }
          frame True {
            n786 = Not(x=w1154) -> (.not. x?=w1153:bool)
            n787 = local write "LIVE FEED MIN TEMP"(w1153) -> ()
            n788 = call "CAMERA LIVE FEED FGV.vi"("Enum - Menu"=CAMERA_LIVE_FEED_ENUM."CAMERA MINIMIZE") -> ()  [unwired: 9 in, 2 out]
          }
        }
        n789 = local write "CAMERA ROI MAX TEMP"(TRUE ("CAMERA ROI MAX TEMP")) -> ()
        n790 = case shown="True" w1145 {
          selector: w1145 -> [_ w1151]
          frame False {
          }
          frame True {
            n791 = Not(x=w1151) -> (.not. x?=w1150:bool)
            n792 = local write "CAMERA ROI MIN TEMP"(w1150) -> ()
            n793 = call "IMAGE ANALYSIS.vi"("Enum"=POST_ANALYSIS_ENUM."MINIMIZE UI") -> ()  [unwired: 9 in, 2 out]
          }
        }
      }
    }
    n794 = local read "Auto Start Test"() -> (w909:bool)
    n795 = case shown="True" "sign in temp" {
      frame False {
      }
      frame True {
        w946 = 1 ("y")
        n796 = local read "USERNAME"() -> (w952:string)
        n797 = local read "USER ID"() -> (w949:string)
        n798 = call <vilib>:"Trim Whitespace.vi"("string"=w952) -> ("trimmed string"=w951:string)  [unwired: 1 in]
        n799 = call <vilib>:"Trim Whitespace.vi"("string"=w949) -> ("trimmed string"=w950:string)  [unwired: 1 in]
        n800 = String Length(string=w951) -> (length=w948:i32)
        n801 = String Length(string=w950) -> (length=w947:i32)
        n802 = Greater?(x=w948, y=w946) -> (0:w945:bool)
        n803 = Greater?(x=w947, y=w946) -> (0:w944:bool)
        n804 = And(x=w945, y=w944) -> (x .and. y?=w943:bool)
        n805 = case shown="True" w943 {
          frame False {
            n806 = property on="Sign In" class="Bool (strict)"("DisabledEnum"=T16."Disabled" ("Disabled")) -> ()  [unwired: 2 in, 2 out]
          }
          frame True {
            n807 = property on="Sign In" class="Bool (strict)"("DisabledEnum"=T16."Enabled" ("Disabled")) -> ()  [unwired: 2 in, 2 out]
          }
        }
      }
    }
    n808 = local read "Air Temperature"() -> (w926:bool)
    n809 = local read "Coefficient Of Friction"() -> (w927:bool)
    n810 = case shown="False" w909 {
      frame False {
        n811 = local read "Auto stop temp"() -> (w940:bool)
        n812 = case shown="True" w940 {
          frame False {
          }
          frame True {
            n813 = local write "Auto Start Temp"(FALSE ("Auto Start Temp")) -> ()
          }
        }
      }
      frame True {
        "Auto stop temp" <- TRUE ("Auto stop temp")
      }
    }
    n814 = local read "Humidity"() -> (w925:bool)
    n815 = case shown="\"HOME\"" w937 {
      frame "HOME" {
        n816 = local write "main tab sub"(enum32{"Page 1", "Page 2"}."Page 1" ("main tab sub")) -> ()
      }
      frame Default {
        n817 = local write "main tab sub"(enum32{"Page 1", "Page 2"}."Page 2" ("main tab sub")) -> ()
      }
    }
    n818 = case shown="True" w936 {
      selector: w936 -> [_ w1259]
      frame False {
      }
      frame True {
        n819 = Not(x=w1259) -> (.not. x?=w1258:bool)
        n820 = local write "Sign In"(w1258) -> ()
        n821 = local write "Main Dashboard Buttons"(T1."Test Setup" ("Main Dashboard Buttons")) -> ()
      }
    }
    n822 = case shown="\"Numeric Display\", Default" "Num/Graph" {
      frame "Numeric Display", Default {
        n823 = property on="Single/Multiple" class="RadioBtnsControl (strict)"("Visible"=FALSE) -> ()  [unwired: 2 in, 2 out]
        n824 = property on="Single - Graph" class="Ring (strict)"("Visible"=FALSE) -> ()  [unwired: 2 in, 2 out]
        n825 = local write "Main Tab Display"(T4."Dashboard 1" ("Main Tab Display")) -> ()
      }
      frame "Graph Display" {
        n826 = property on="Single/Multiple" class="RadioBtnsControl (strict)"("Visible"=TRUE) -> ()  [unwired: 2 in, 2 out]
        n827 = case shown="\"Multiple\"" "Single/Multiple" {
          frame "Single ", Default {
            n828 = property on="Single - Graph" class="Ring (strict)"("Visible"=TRUE) -> ()  [unwired: 2 in, 2 out]
            n829 = local write "Main Tab Display"(T4."Dashboard 3" ("Main Tab Display")) -> ()
          }
          frame "Multiple" {
            n830 = property on="Single - Graph" class="Ring (strict)"("Visible"=FALSE) -> ()  [unwired: 2 in, 2 out]
            n831 = local write "Main Tab Display"(T4."Dashboard 2" ("Main Tab Display")) -> ()
          }
        }
      }
    }
    n832 = local read "Stroke"() -> (w924:bool)
    n833 = local read "USERNAME"() -> (w930:string)
    n834 = local read "USER ID"() -> (w929:string)
    n835 = case shown="True" w927 {
      selector: w927 -> [_ w1194]
      frame False {
      }
      frame True {
        n836 = Not(x=w1194) -> (.not. x?=w1193:bool)
        n837 = local write "Coefficient Of Friction"(w1193) -> ()
        n838 = local write "Tab Control 2"(T6."Coefficient Of Friction" ("Tab Control 2")) -> ()
      }
    }
    n839 = case shown="True" w926 {
      selector: w926 -> [_ w1191]
      frame False {
      }
      frame True {
        n840 = Not(x=w1191) -> (.not. x?=w1189:bool)
        n841 = local write "Air Temperature"(w1189) -> ()
        n842 = local write "Tab Control 2"(T6."Air Temperature" ("Tab Control 2")) -> ()
      }
    }
    n843 = local write "Operator ID"(w929) -> ()
    n844 = case shown="True" w924 {
      selector: w924 -> [_ w1185]
      frame False {
      }
      frame True {
        n845 = Not(x=w1185) -> (.not. x?=w1183:bool)
        n846 = local write "Stroke"(w1183) -> ()
        n847 = local write "Tab Control 2"(T6."Stroke" ("Tab Control 2")) -> ()
      }
    }
    n848 = local write "tested by"(w930) -> ()
    n849 = case shown="True" w925 {
      selector: w925 -> [_ w1188]
      frame False {
      }
      frame True {
        n850 = Not(x=w1188) -> (.not. x?=w1186:bool)
        n851 = local write "Humidity"(w1186) -> ()
        n852 = local write "Tab Control 2"(T6."Humidity" ("Tab Control 2")) -> ()
      }
    }
    n853 = case shown="\"Advance\"" "Main Dashboard Buttons" {
      tunnel: [T2."HOME" ("Main Tab") T2."Test Setup" ("Main Tab") T2."Acquire" ("Main Tab") T2."Adv Scar" ("Main Tab") T2."Adv Scar Report" ("Main Tab") T2."Compare Files" ("Main Tab") T2."About" ("Main Tab") T2."Advance" ("Main Tab")] -> w934
      frame "Home", Default {
      }
      frame "Test Setup" {
      }
      frame "Dashboard" {
      }
      frame "Imaging" {
      }
      frame "Report" {
      }
      frame "Analysis" {
      }
      frame "About" {
      }
      frame "Advance" {
      }
    }
    n854 = Wait (ms)(milliseconds to wait=u32 100) -> ()  [unwired: 1 out]
    n855 = local read "Main Tab Display"() -> (w928:T4)
    n856 = local write "Main Tab"(w934) -> ()
    n857 = case shown="\"Dashboard 3\"" w928 {
      frame "Dashboard 1", Default {
        n858 = property on="Reset Graph" class="Bool (strict)"("Visible"=FALSE) -> ()  [unwired: 2 in, 2 out]
      }
      frame "Dashboard 2" {
        n859 = property on="Reset Graph" class="Bool (strict)"("Visible"=TRUE) -> ()  [unwired: 2 in, 2 out]
      }
      frame "Dashboard 3" {
        n860 = property on="Reset Graph" class="Bool (strict)"("Visible"=TRUE) -> ()  [unwired: 2 in, 2 out]
      }
    }
    n861 = local read "SCAR MEASURMENT"() -> (w916:enum32{"Auto Scar", "Manual Scar"})
    n862 = local read "Humidity"() -> (w931:bool)
    n863 = local read "Cap Live Image"() -> (w913:bool)
    n864 = local read "Sample Temperature"() -> (w923:bool)
    n865 = local read "Air Temp vs Humidity"() -> (w921:bool)
    n866 = local read "Frequency"() -> (w922:bool)
    n867 = case shown="False" w931 {
      frame False {
        n868 = local write "Humidity On Command"(TRUE ("Humidity On Command")) -> ()
        n869 = case shown="True" "Humidity Off Command" {
          selector: "Humidity Off Command" -> [_ w1201]
          frame False {
          }
          frame True {
            n870 = stacked-sequence {
              frame #0 {
                n871 = local read "WriteHumidity"() -> (w1203:string[])
                n872 = Insert Into Array(array=w1203, new element="R;1" ("new element/subarray")) -> (w1204:string[])  [unwired: 1 in]
                n873 = local write "WriteHumidity"(w1204) -> ()
              }
              frame #1 {
                n874 = Wait (ms)(milliseconds to wait=u32 2000) -> ()  [unwired: 1 out]
              }
              frame #2 {
                n875 = local read "EVENT LOG"() -> (w1210:string)
                n876 = local read "WriteHumidity"() -> (w1207:string[])
                n877 = call "Event Log.vi"("Content"="Humidity Control Off" ("string"), "EVENT LOG"=w1210) -> ("EVENT LOG"=w1211:string)  [unwired: 8 in, 1 out]
                n878 = local write "EVENT LOG"(w1211) -> ()
                n879 = Insert Into Array(array=w1207, new element="R;1" ("new element/subarray")) -> (w1208:string[])  [unwired: 1 in]
                n880 = local write "WriteHumidity"(w1208) -> ()
              }
            }
            n881 = Not(x=w1201) -> (.not. x?=w1200:bool)
            n882 = local write "Humidity Off Command"(w1200) -> ()
          }
        }
      }
      frame True {
        n883 = local write "Humidity Off Command"(TRUE ("Humidity Off Command")) -> ()
        n884 = case shown="False" "Humidity On Command" {
          selector: "Humidity On Command" -> [_ w1215]
          frame False {
          }
          frame True {
            n885 = stacked-sequence {
              frame #0 {
                n886 = local read "Set Rh"() -> (w1221:dbl)
                n887 = Number To Fractional String(number=w1221, precision (6)=i16 2) -> (F-format string=w1222:string)  [unwired: 2 in]
                n888 = local read "WriteHumidity"() -> (w1219:string[])
                n889 = Concatenate Strings("M;" ("new element/subarray"), w1222) -> (w1220:string)
                n890 = Insert Into Array(array=w1219, new element=w1220) -> (w1218:string[])  [unwired: 1 in]
                n891 = local write "WriteHumidity"(w1218) -> ()
              }
              frame #1 {
                n892 = Wait (ms)(milliseconds to wait=u32 1500) -> ()  [unwired: 1 out]
              }
              frame #2 {
                (unwired) "% RH" ("string")
                (unwired) i16 2 ("precision (6)")
                (unwired) "M;" ("new element/subarray")
                n893 = local read "Set Rh"() -> (w1229:dbl)
                n894 = Number To Fractional String(number=w1229, precision (6)=i16 2) -> (F-format string=w1226:string)  [unwired: 2 in]
                n895 = local read "WriteHumidity"() -> (w1231:string[])
                n896 = Concatenate Strings("M;" ("new element/subarray"), w1226) -> (w1230:string)
                n897 = Concatenate Strings("Humidity Set to : " ("string"), w1226, "% RH" ("string")) -> (w1224:string)
                n898 = Insert Into Array(array=w1231, new element=w1230) -> (w1232:string[])  [unwired: 1 in]
                n899 = disable-structure shown="Enabled" {
                  frame Enabled {
                    n900 = local read "EVENT LOG"() -> (w1235:string)
                    n901 = call "Event Log.vi"("Content"="Humidity Control On", "EVENT LOG"=w1235) -> ("EVENT LOG"=w1236:string)  [unwired: 8 in, 1 out]
                    n902 = local write "EVENT LOG"(w1236) -> ()
                  }
                  frame Disabled {
                  }
                }
                n903 = disable-structure shown="Enabled" {
                  disable-tunnel: w1224 -> [_ _]
                  frame Enabled {
                    n904 = local read "EVENT LOG"() -> (w1238:string)
                    n905 = call "Event Log.vi"("Content"="Humidity Control On", "EVENT LOG"=w1238) -> ("EVENT LOG"=w1239:string)  [unwired: 8 in, 1 out]
                    n906 = local write "EVENT LOG"(w1239) -> ()
                  }
                  frame Disabled {
                  }
                }
                n907 = local write "WriteHumidity"(w1232) -> ()
              }
            }
            n908 = Not(x=w1215) -> (.not. x?=w1214:bool)
            n909 = local write "Humidity On Command"(w1214) -> ()
          }
        }
      }
    }
    n910 = Equal?(x=w916, y=enum32{"Auto Scar", "Manual Scar"}."Auto Scar" ("SCAR MEASURMENT")) -> (x = y?=w912:bool)
    n911 = local read "TEST STANDARD"() -> (w919:T3)
    n912 = And(x=w913, y=w912) -> (x .and. y?=w914:bool)
    n913 = case shown="True" w914 {
      selector: w914 -> [_ w1013]
      tunnel: errorcluster {"status"=FALSE, "code"=0, "source"=""} ("error in (no error) 3") -> [_ w1014]
      frame False {
      }
      frame True {
        n914 = stacked-sequence {
          tunnel: w1014 -> [_ _ _ _ _ _ _ w1058]
          tunnel: w1013 -> [_ _ _ _ _ w1041 _ _]
          frame #0 {
            n915 = call "CAMERA LIVE FEED FGV.vi"("Enum - Menu"=CAMERA_LIVE_FEED_ENUM."CAMERA MINIMIZE") -> ()  [unwired: 9 in, 2 out]
          }
          frame #1 {
            n916 = property on="Auto Scar Check  2" class="Clust (strict)"("Visible"=TRUE) -> ()  [unwired: 2 in, 2 out]
          }
          frame #2 {
            n917 = String To Path(string="C:\\LAB-IQ\\Image Calibrate v01.dcf") -> (path=w1019:path)
            n918 = Open/Create/Replace File ("Open File")(file path (use dialog)=w1019) -> (refnum out=w1020:refnum<file>)  [unwired: 5 in, 2 out]
            n919 = for {
              N: 4 -> [_]
              tunnel: w1020 -> [w1026]
              i -> [w1022]
              n920 = Read from Text File ("Read File")(file (use dialog)=w1026) -> (text=w1027:string)  [unwired: 3 in, 3 out]
              n921 = String Subset(string=w1027, offset (0)=6, length (rest)=10 ("length (rest)")) -> (substring=w1023:string)
              n922 = Fract/Exp String To Number(string=w1023) -> (number=w1021:dbl)  [unwired: 3 in, 1 out]
              n923 = case shown="0" w1022 {
                tunnel: w1021 -> [w1028 w1029 _ w1030 _]
                frame 0 {
                  "5x Gain" <- w1028
                }
                frame 1 {
                  "10x Gain" <- w1029
                }
                frame 2 {
                }
                frame 3 {
                  "100x gain" <- w1030
                }
                frame 4, Default {
                }
              }
            }
          }
          frame #3 {
            n924 = local read "FILE 3"() -> (w1036:string)
            n925 = call <vilib>:"Trim Whitespace.vi"("string"="C:\\LAB-IQ\\images\\") -> ("trimmed string"=w1038:string)  [unwired: 1 in]
            n926 = String To Path(string=w1038) -> (path=w1037:path)
            n927 = Concatenate Strings(w1036, ".png" ("string")) -> (w1035:string)
            n928 = Build Path(base path=w1037, name or relative path=w1035) -> (appended path=w1033:path)
            "Image path" <- w1033
            n929 = Path To String(path=w1033) -> (string=w1032:string)
            n930 = call "CAMERA LIVE FEED FGV.vi"("Enum - Menu"=CAMERA_LIVE_FEED_ENUM."CAMERA SAVE", "Image Path"=w1032) -> ()  [unwired: 8 in, 2 out]
          }
          frame #4 {
            n931 = One Button Dialog(message="Image saved successfully") -> ()  [unwired: 1 in, 1 out]
          }
          frame #5 {
            n932 = local read "Magnification len live scar"() -> (w1052:string)
            n933 = Not(x=w1041) -> (.not. x?=w1042:bool)
            n934 = local write "Cap Live Image"(w1042) -> ()
            n935 = case shown="\"5x\", Default" w1052 {
              tunnel: [w1053 w1054] -> w1051
              frame "5x", Default {
                n936 = local read "5x Gain"() -> (w1053:dbl)
              }
              frame "10x" {
                # "5x"
                n937 = local read "10x Gain"() -> (w1054:dbl)
              }
            }
            n938 = local read "Image path"() -> (w1050:path)
            n939 = local read "FILE 3"() -> (w1043:string)
            n940 = call "EDGE DETCTION.vi"("GAIN VALUE"=w1051, "Image Path"=w1050) -> ("error out"=w1049:errorcluster, "return value"=w1048:cluster{string, string, dbl, dbl, dbl})  [unwired: 8 in]
            n941 = Bundle By Name(cluster=T21 {"File Name"="", "Test Method"="", "Operator"="", "Fuel Description"="", "Date and time"=""} ("Main Ref"), "File Name"=w1043) -> (w1044:T21)
            n942 = call "duf file read.vi"("error in (no error)"=w1049, "Main Ref"=w1044) -> ("error out"=w1047:errorcluster, "Main Ref 2"=w1045:T21)  [unwired: 8 in]
            n943 = call "EDGE DETECTION REPORT.vi"("error in (no error)"=w1047, "return value 2"=w1048, "Main Ref"=w1045) -> ()  [unwired: 8 in, 1 out]
          }
          frame #6 {
            n944 = property on="Auto Scar Check  2" class="Clust (strict)"("Visible"=FALSE) -> ()  [unwired: 2 in, 2 out]
          }
          frame #7 {
            n945 = call "CAMERA LIVE FEED FGV.vi"("Enum - Menu"=CAMERA_LIVE_FEED_ENUM."CAMERA MINIMIZE", "error in (no error)"=w1058) -> ()  [unwired: 8 in, 2 out]
            n946 = local write "Main Dashboard Buttons"(T1."Home" ("Main Dashboard Buttons")) -> ()
            n947 = local write "Main Tab"(T2."HOME" ("Main Tab")) -> ()
          }
        }
      }
    }
    n948 = local read "Heater Button"() -> (w920:bool)
    n949 = case shown="True" w922 {
      selector: w922 -> [_ w1179]
      frame False {
      }
      frame True {
        n950 = Not(x=w1179) -> (.not. x?=w1177:bool)
        n951 = local write "Frequency"(w1177) -> ()
        n952 = local write "Tab Control 2"(T6."Frequency" ("Tab Control 2")) -> ()
      }
    }
    n953 = case shown="True" w921 {
      selector: w921 -> [_ w1176]
      frame False {
      }
      frame True {
        n954 = Not(x=w1176) -> (.not. x?=w1174:bool)
        n955 = local write "Air Temp vs Humidity"(w1174) -> ()
        n956 = local write "Tab Control 2"(T6."Air Temp vs Rh" ("Tab Control 2")) -> ()
      }
    }
    n957 = case shown="True" w923 {
      selector: w923 -> [_ w1182]
      frame False {
      }
      frame True {
        n958 = Not(x=w1182) -> (.not. x?=w1180:bool)
        n959 = local write "Sample Temperature"(w1180) -> ()
        n960 = local write "Tab Control 2"(T6."Sample Temperature" ("Tab Control 2")) -> ()
      }
    }
    n961 = case shown="\"Custom\"" w919 {
      frame "ASTM D6079", Default {
        w1155 = "ASTM D6079 TEST CONDITIONS" ("Standard 2")
        n962 = local write "Standard 2"(w1155) -> ()
        n963 = local write "Standard"(w1155) -> ()
      }
      frame "ISO 12156" {
        w1156 = "ISO 12156 TEST CONDITIONS" ("Standard 2")
        n964 = local write "Standard 2"(w1156) -> ()
        n965 = local write "Standard"(w1156) -> ()
      }
      frame "CEC F-096-A-06" {
        w1157 = "CEC F-096-A-06 TEST CONDITIONS" ("Standard 2")
        n966 = local write "Standard 2"(w1157) -> ()
        n967 = local write "Standard"(w1157) -> ()
      }
      frame "Custom" {
        w1158 = "CUSTOM TEST CONDITIONS" ("Standard 2")
        n968 = local write "Standard 2"(w1158) -> ()
        n969 = local write "Standard"(w1158) -> ()
      }
    }
    n970 = case shown="True" w920 {
      frame False {
        n971 = local write "Temperature On Command"(TRUE ("Temperature On Command")) -> ()
        n972 = case shown="True" "Temperature Off Command" {
          selector: "Temperature Off Command" -> [_ w1162]
          frame False {
          }
          frame True {
            n973 = Not(x=w1162) -> (.not. x?=w1161:bool)
            n974 = local read "EVENT LOG"() -> (w1165:string)
            n975 = local write "Temperature Off Command"(w1161) -> ()
            n976 = call "Event Log.vi"("Content"="Heater Off", "EVENT LOG"=w1165) -> ("EVENT LOG"=w1164:string)  [unwired: 8 in, 1 out]
            n977 = local write "EVENT LOG"(w1164) -> ()
          }
        }
      }
      frame True {
        n978 = local write "Temperature Off Command"(TRUE ("Temperature Off Command")) -> ()
        n979 = case shown="True" "Temperature On Command" {
          selector: "Temperature On Command" -> [_ w1169]
          frame False {
          }
          frame True {
            n980 = Not(x=w1169) -> (.not. x?=w1168:bool)
            n981 = local write "Temperature On Command"(w1168) -> ()
            n982 = disable-structure shown="Enabled" {
              disable-tunnel: "Heater On" -> [w1171 _]
              frame Enabled {
                n983 = local read "EVENT LOG"() -> (w1172:string)
                n984 = call "Event Log.vi"("Content"=w1171, "EVENT LOG"=w1172) -> ("EVENT LOG"=w1173:string)  [unwired: 8 in, 1 out]
                n985 = local write "EVENT LOG"(w1173) -> ()
              }
              frame Disabled {
              }
            }
          }
        }
      }
    }
    n986 = local read "Main Tab"() -> (w911:T2)
    n987 = case shown="\"About\"" w911 {
      frame "HOME", Default {
        w957 = T16."Enabled" ("Disabled")
        n988 = local read "Service Password enable"() -> (w956:bool)
        n989 = property on="Imaging" class="Bool (strict)"("DisabledEnum"=w957) -> ()  [unwired: 2 in, 2 out]
        n990 = property on="Dashboard" class="Bool (strict)"("DisabledEnum"=w957) -> ()  [unwired: 2 in, 2 out]
        n991 = property on="Test Setup" class="Bool (strict)"("DisabledEnum"=w957) -> ()  [unwired: 2 in, 2 out]
        n992 = property on="Analysis" class="Bool (strict)"("DisabledEnum"=w957) -> ()  [unwired: 2 in, 2 out]
        n993 = property on="Home" class="Bool (strict)"("DisabledEnum"=w957) -> ()  [unwired: 2 in, 2 out]
        n994 = property on="Report" class="Bool (strict)"("DisabledEnum"=w957) -> ()  [unwired: 2 in, 2 out]
        n995 = property on="Main Dashboard Buttons" class="RadioBtnsControl (strict)"("DisabledEnum"=w957) -> ()  [unwired: 2 in, 2 out]
        n996 = case shown="True" w956 {
          tunnel: [T16."Disabled" ("Disabled") T16."Enabled" ("Disabled")] -> w955
          frame False {
          }
          frame True {
          }
        }
        n997 = property on="About" class="Bool (strict)"("DisabledEnum"=w955) -> ()  [unwired: 2 in, 2 out]
      }
      frame "Test Setup" {
        w962 = T16."Enabled" ("Disabled")
        n998 = local read "Service Password enable"() -> (w961:bool)
        n999 = property on="Dashboard" class="Bool (strict)"("DisabledEnum"=T16."Disabled" ("Disabled")) -> ()  [unwired: 2 in, 2 out]
        n1000 = property on="Imaging" class="Bool (strict)"("DisabledEnum"=w962) -> ()  [unwired: 2 in, 2 out]
        n1001 = property on="Analysis" class="Bool (strict)"("DisabledEnum"=w962) -> ()  [unwired: 2 in, 2 out]
        n1002 = property on="Home" class="Bool (strict)"("DisabledEnum"=w962) -> ()  [unwired: 2 in, 2 out]
        n1003 = property on="Report" class="Bool (strict)"("DisabledEnum"=w962) -> ()  [unwired: 2 in, 2 out]
        n1004 = property on="Test Setup" class="Bool (strict)"("DisabledEnum"=w962) -> ()  [unwired: 2 in, 2 out]
        n1005 = case shown="True" w961 {
          tunnel: [T16."Disabled" ("Disabled") T16."Enabled" ("Disabled")] -> w960
          frame False {
          }
          frame True {
          }
        }
        n1006 = property on="About" class="Bool (strict)"("DisabledEnum"=w960) -> ()  [unwired: 2 in, 2 out]
      }
      frame "Adv Scar" {
        w969 = T16."Enabled" ("Disabled")
        n1007 = property on="Dashboard" class="Bool (strict)"("DisabledEnum"=T16."Disabled" ("Disabled")) -> ()  [unwired: 2 in, 2 out]
        n1008 = property on="Imaging" class="Bool (strict)"("DisabledEnum"=w969) -> ()  [unwired: 2 in, 2 out]
